vi "Start.vi"(8 "error in (no error)":errorcluster, 11 "Module Config Selector":i16) -> (0 "error out":errorcluster)   [LabVIEW 2017, in "VDMS_VibAPI_8.lvlib"]
uses:
  <vilib>/addons/InsightCM/Devices/Shared/Cms/Fpga/AcquisitionFpgaTach/source/subVIs/VibAPI_8/VDMS_VibAPI_8.lvlib
  <vilib>/rvi/eio/common/nirviEmuTemplateMethod_errors.vi
  <vilib>/eio/EIONode/EIONode.xnode
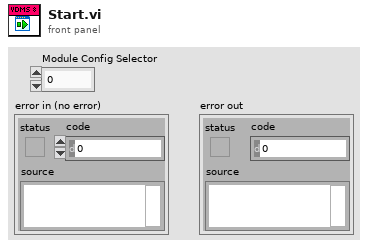
[diagram p1: front panel]
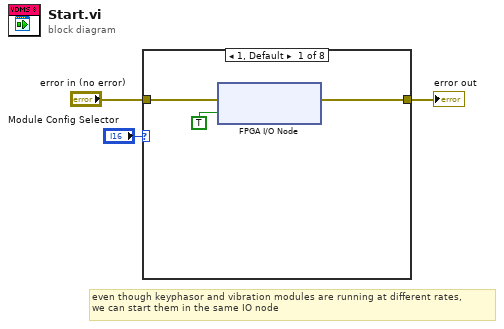
[diagram p0: block diagram]
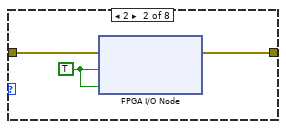
[diagram p2: hidden frame]
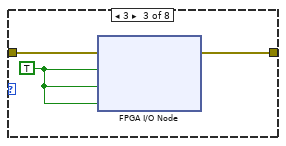
[diagram p3: hidden frame]
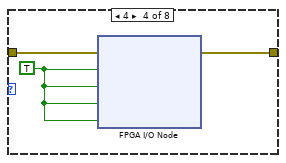
[diagram p4: hidden frame]
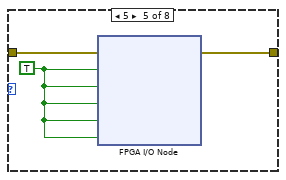
[diagram p5: hidden frame]
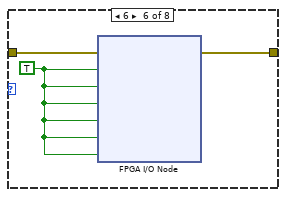
[diagram p6: hidden frame]
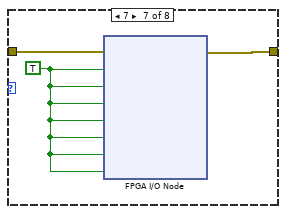
[diagram p7: hidden frame]
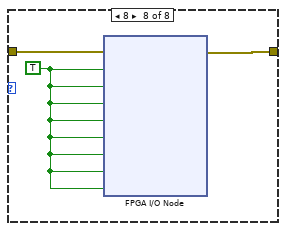
[diagram p8: hidden frame]
diagram:
  # "even though keyphasor and vibration modules are running at different rates,\nwe can start them in the same IO node"
  n1 = case shown="1, Default" "Module Config Selector" {
    tunnel: "error in (no error)" -> [w5 w8 w12 w15 w18 w21 w24 w27]
    tunnel: [w6 w9 w10 w14 w17 w20 w23 w26] -> w2
    frame 1, Default {
      n2 = xnode "FPGA I/O Node"("error in"=w5, "Mod1/Start"=TRUE) -> ("error out"=w6:errorcluster)  [unwired: 1 in, 1 out]
    }
    frame 2 {
      w7 = TRUE
      n3 = xnode "FPGA I/O Node"("error in"=w8, "Mod1/Start"=w7, "Mod2/Start"=w7) -> ("error out"=w9:errorcluster)  [unwired: 2 in, 2 out]
    }
    frame 3 {
      w11 = TRUE ("Mod1/Start")
      n4 = xnode "FPGA I/O Node"("error in"=w12, "Mod1/Start"=w11, "Mod2/Start"=w11, "Mod3/Start"=w11) -> ("error out"=w10:errorcluster)  [unwired: 3 in, 3 out]
    }
    frame 4 {
      w13 = TRUE ("Mod1/Start")
      n5 = xnode "FPGA I/O Node"("error in"=w15, "Mod1/Start"=w13, "Mod2/Start"=w13, "Mod3/Start"=w13, "Mod4/Start"=w13) -> ("error out"=w14:errorcluster)  [unwired: 4 in, 4 out]
    }
    frame 5 {
      w16 = TRUE ("Mod1/Start")
      n6 = xnode "FPGA I/O Node"("error in"=w18, "Mod1/Start"=w16, "Mod2/Start"=w16, "Mod3/Start"=w16, "Mod4/Start"=w16, "Mod5/Start"=w16) -> ("error out"=w17:errorcluster)  [unwired: 5 in, 5 out]
    }
    frame 6 {
      w19 = TRUE ("Mod1/Start")
      n7 = xnode "FPGA I/O Node"("error in"=w21, "Mod1/Start"=w19, "Mod2/Start"=w19, "Mod3/Start"=w19, "Mod4/Start"=w19, "Mod5/Start"=w19, "Mod6/Start"=w19) -> ("error out"=w20:errorcluster)  [unwired: 6 in, 6 out]
    }
    frame 7 {
      w22 = TRUE ("Mod1/Start")
      n8 = xnode "FPGA I/O Node"("error in"=w24, "Mod1/Start"=w22, "Mod2/Start"=w22, "Mod3/Start"=w22, "Mod4/Start"=w22, "Mod5/Start"=w22, "Mod6/Start"=w22, "Mod7/Start"=w22) -> ("error out"=w23:errorcluster)  [unwired: 7 in, 7 out]
    }
    frame 8 {
      w25 = TRUE ("Mod1/Start")
      n9 = xnode "FPGA I/O Node"("error in"=w27, "Mod1/Start"=w25, "Mod2/Start"=w25, "Mod3/Start"=w25, "Mod4/Start"=w25, "Mod5/Start"=w25, "Mod6/Start"=w25, "Mod7/Start"=w25, "Mod8/Start"=w25) -> ("error out"=w26:errorcluster)  [unwired: 8 in, 8 out]
    }
  }
  "error out" <- w2
